vi "Global_Buffer.vi"() -> ()   [LabVIEW 2023]
panel:
  out "Vitesse Z":dbl
  out "Vitesse Y":dbl
  out "Vitesse X":dbl
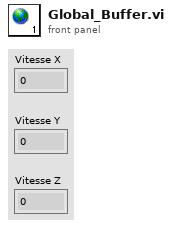
[diagram p1: front panel]
diagram:
